vi "Calculate run moves.vi"(7 "Position":refnum<class "Position.lvclass">, 9 "Direction":T1, 10 "Source":T2={"File"=enum."d", "Rank"=enum."4"}, 11 "Runner in":refnum<class "Runner.lvclass">) -> (2 "Moves":refnum<class "Move.lvclass">[](array[class]), 3 "Runner out":refnum<class "Runner.lvclass">)   [LabVIEW 2016, in "Chesslib.lvlib" / "Runner.lvclass"]
uses:
  Runner.lvclass
  C:/Users/GRTaggJ/Documents/Projects/checkmate/Chesslib/Pieces/Piece/Piece.lvclass
  typedef/Square.ctl
  typedef/File.ctl
  typedef/Rank.ctl
  Position/Position.lvclass
  Moves/Move/Move.lvclass
  typedef/Direction.ctl
  typedef/Neighbor.ctl
  Chesslib.lvlib
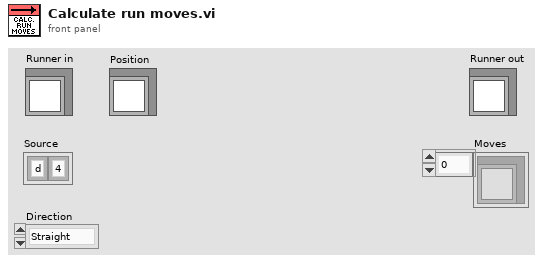
[diagram p1: front panel]
types:
  T1 = typedef "Chesslib.lvlib/Direction.ctl" = enum16{"Straight", "Diagonal", "Both"}
  T2 = typedef "Chesslib.lvlib/Square.ctl" = cluster{"File":T3, "Rank":T4}
  T3 = typedef "Chesslib.lvlib/File.ctl" = enum8{"a", "b", "c", "d", "e", "f", "g", "h"}
  T4 = typedef "Chesslib.lvlib/Rank.ctl" = enum8{"1", "2", "3", "4", "5", "6", "7", "8"}
  T5 = typedef "Chesslib.lvlib/Neighbor.ctl" = enum16{"N", "NW", "W", "SW", "S", "SE", "E", "NE"}
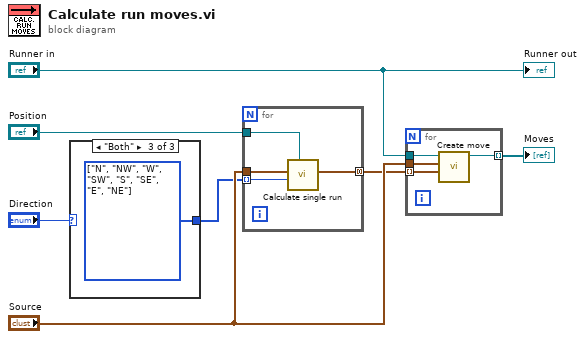
[diagram p0: block diagram]
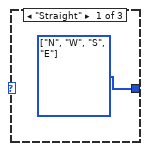
[diagram p2: hidden frame]
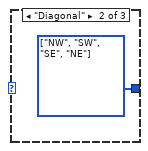
[diagram p3: hidden frame]
diagram:
  n1 = case shown="\"Both\"" "Direction" {
    tunnel: [w8 w9 w10] -> w3
    frame "Straight" {
      w8 = T5[] [enum."N", enum."W", enum."S", enum."E"] items=["N", "NW", "W", "SW", "S", "SE", "E", "NE"]
    }
    frame "Diagonal" {
      w9 = T5[] [enum."NW", enum."SW", enum."SE", enum."NE"] items=["N", "NW", "W", "SW", "S", "SE", "E", "NE"]
    }
    frame "Both" {
      w10 = T5[] [enum."N", enum."NW", enum."W", enum."SW", enum."S", enum."SE", enum."E", enum."NE"] items=["N", "NW", "W", "SW", "S", "SE", "E", "NE"]
    }
  }
  n2 = for {
    tunnel: "Position" -> [w14]
    tunnel: "Source" -> [w13]
    tunnel: w3 -> [w12] mode=indexing
    tunnel: [w11] -> w2 mode=concatenating
    n3 = call "Calculate single run.vi"("Board"=w14, "Direction"=w12, "Source"=w13) -> ("Destinations"=w11:T2[])  [unwired: 8 in]
  }
  n4 = for {
    tunnel: w2 -> [w18] mode=indexing
    tunnel: [w17] -> w4 mode=indexing
    tunnel: "Source" -> [w16]
    tunnel: "Runner in" -> [w15]
    n5 = call "Create move.vi"("Destination"=w18, "Source"=w16, "Piece"=w15) -> ("Move out"=w17:refnum<class "Move.lvclass">)  [unwired: 8 in]
  }
  "Moves" <- w4
  "Runner out" <- "Runner in"
